vi "Autonomous Independent.vi"() -> ()   [LabVIEW 2015]
doc: "This VI is called when autonomous begins, and will automatically be terminated when autonomous ends. You can carry out timed or sensor driven robot movement independently without needing to return to the caller."
uses:
  <vilib>/Rock Robotics/WPI/Utilities/WPI_GetSetVariantRefNum.vi
  <vilib>/Rock Robotics/Network Tables/NT Write Numeric Array.vi
  <vilib>/Rock Robotics/Network Tables/NT Read Boolean.vi
  <vilib>/Rock Robotics/Network Tables/NT Write Boolean.vi
  <vilib>/Rock Robotics/Network Tables/NT Write Number.vi
  <vilib>/Rock Robotics/Network Tables/NT Read Number.vi
  <vilib>/Rock Robotics/WPI/RobotDrive/WPI_RobotDriveArcadeDrive_Standard(NoSaturation).vi
panel:
  in  "Ticks to Turn":i32=36
  out "VAR-Storage-1":dbl
  out "Low Switch":bool
  out "High Switch":bool
  out "POT Sensor Meter":dbl(knob) scale=78.0..98.0
  out "POT Sensor Value":dbl
  # "Remeber to Right Click:\nData Operatoins -> Make Current Value Default"
  # "Also This value is the \nTotal amount of ticks not Turns!\n\nSo 6 Ticks EQU 1 Full Turn."
  # "Be sure to right-click and choose Data Operations>>Make Current Value default if you want to save the array values with the VI"
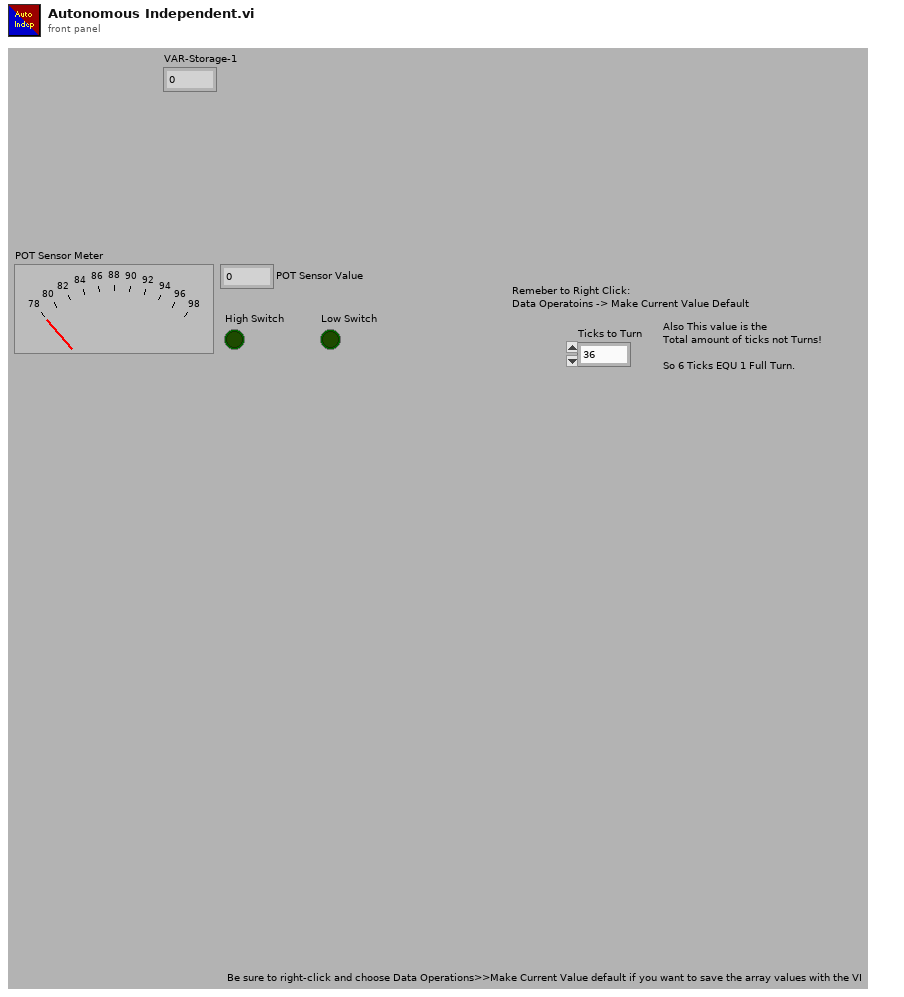
[diagram p1: front panel]
types:
  T1 = typedef "WPI_JoystickDevRef.ctl" = cluster{"Device":T2}
  T2 = typedef "WPI_JoystickDeviceEnum.ctl" = enum16{"USB 0", "USB 1", "USB 2", "USB 3", "USB 4", "USB 5"}
  T3 = typedef "WPI_CounterDevRef.ctl" = cluster{"DevStatus":errorcluster, "CntIndex":T4}
  T4 = typedef "FPGA_CounterCtrSystemIndex.ctl" = enum8{"Ctr 0", "Ctr 1", "Ctr 2", "Ctr 3", "Ctr 4", "Ctr 5", "Ctr 6", "Ctr 7", "Invalid"}
  T5 = typedef "WPI_SwitchDevRef.ctl" = cluster{"DevStatus":errorcluster, "DIO Channel":T6, "CntIndex":T4, "Normally Closed":bool}
  T6 = typedef "FPGA_DIOChannel.ctl" = enum8{"DIO 0", "DIO 1", "DIO 2", "DIO 3", "DIO 4", "DIO 5", "DIO 6", "DIO 7", "DIO 8", "DIO 9", "DIO MXP 0", "DIO MXP 1", "DIO MXP 2", "DIO MXP 3", "DIO MXP 4", "DIO MXP 5", "DIO MXP 6", "DIO MXP 7", "DIO MXP 8", "DIO MXP 9", "DIO MXP 10", "DIO MXP 11", "DIO MXP 12", "DIO MXP 13", "DIO MXP 14", "DIO MXP 15", "Invalid"}
  T7 = typedef "WPI_PotentiometerDevRef.ctl" = cluster{"DevStatus":errorcluster, "Analog Channel":T8, "Invert Output":bool}
  T8 = typedef "FPGA_AIChannel.ctl" = enum8{"AI 0", "AI 1", "AI 2", "AI 3", "AI MXP 0", "AI MXP 1", "AI MXP 2", "AI MXP 3", "Invalid"}
  T9 = typedef "WPI_MotorControlDeviceRef.ctl" = cluster{"DeviceStatus":errorcluster, "Type":T10, "PWM":cluster{"PWM Channel":T11, "DeadBand":T12}, "CAN":cluster{"Device Number":u8, "Control Mode":T13, "Semaphore":T14, "Max Vout":dbl, "TalonSRX Control Mode":T15}, "Invert":bool}
  T10 = typedef "WPI_MotorControlType.ctl" = enum16{"PWM", "CAN", "CANTalonSRX"}
  T11 = typedef "FPGA_DIOPWMChannel.ctl" = enum8{"PWM 0", "PWM 1", "PWM 2", "PWM 3", "PWM 4", "PWM 5", "PWM 6", "PWM 7", "PWM 8", "PWM 9", "PWM MXP 0", "PWM MXP 1", "PWM MXP 2", "PWM MXP 3", "PWM MXP 4", "PWM MXP 5", "PWM MXP 6", "PWM MXP 7", "PWM MXP 8", "PWM MXP 9", "Invalid"}
  T12 = typedef "WPI_PWMDeadband.ctl" = cluster{"Name":string, "maxPositivePwm":i32, "minPositivePwm":i32, "centerPwm":i32, "maxNegativePwm":i32, "minNegativePwm":i32, "angularRange":u16}
  T13 = typedef "WPI_CANJaguar_ControlMode.ctl" = enum8{"Percent VBus", "Current", "Speed", "Position", "Voltage"}
  T14 = typedef "Semaphore RefNum" = refnum<k1>
  T15 = typedef "WPI_CANTalonSRX_APIControlMode.ctl" = enum8{"Percent VBus", "Speed", "Position", "Slave", "Unchanged / Invalid", "Voltage Compensation", "Current", "Motion Profile"}
  T16 = typedef "WPI_RobotDriveDevRef.ctl" = cluster{"DevStatus":errorcluster, "Motors[]":T9[], "Square Inputs":bool, "Max Output":dbl}
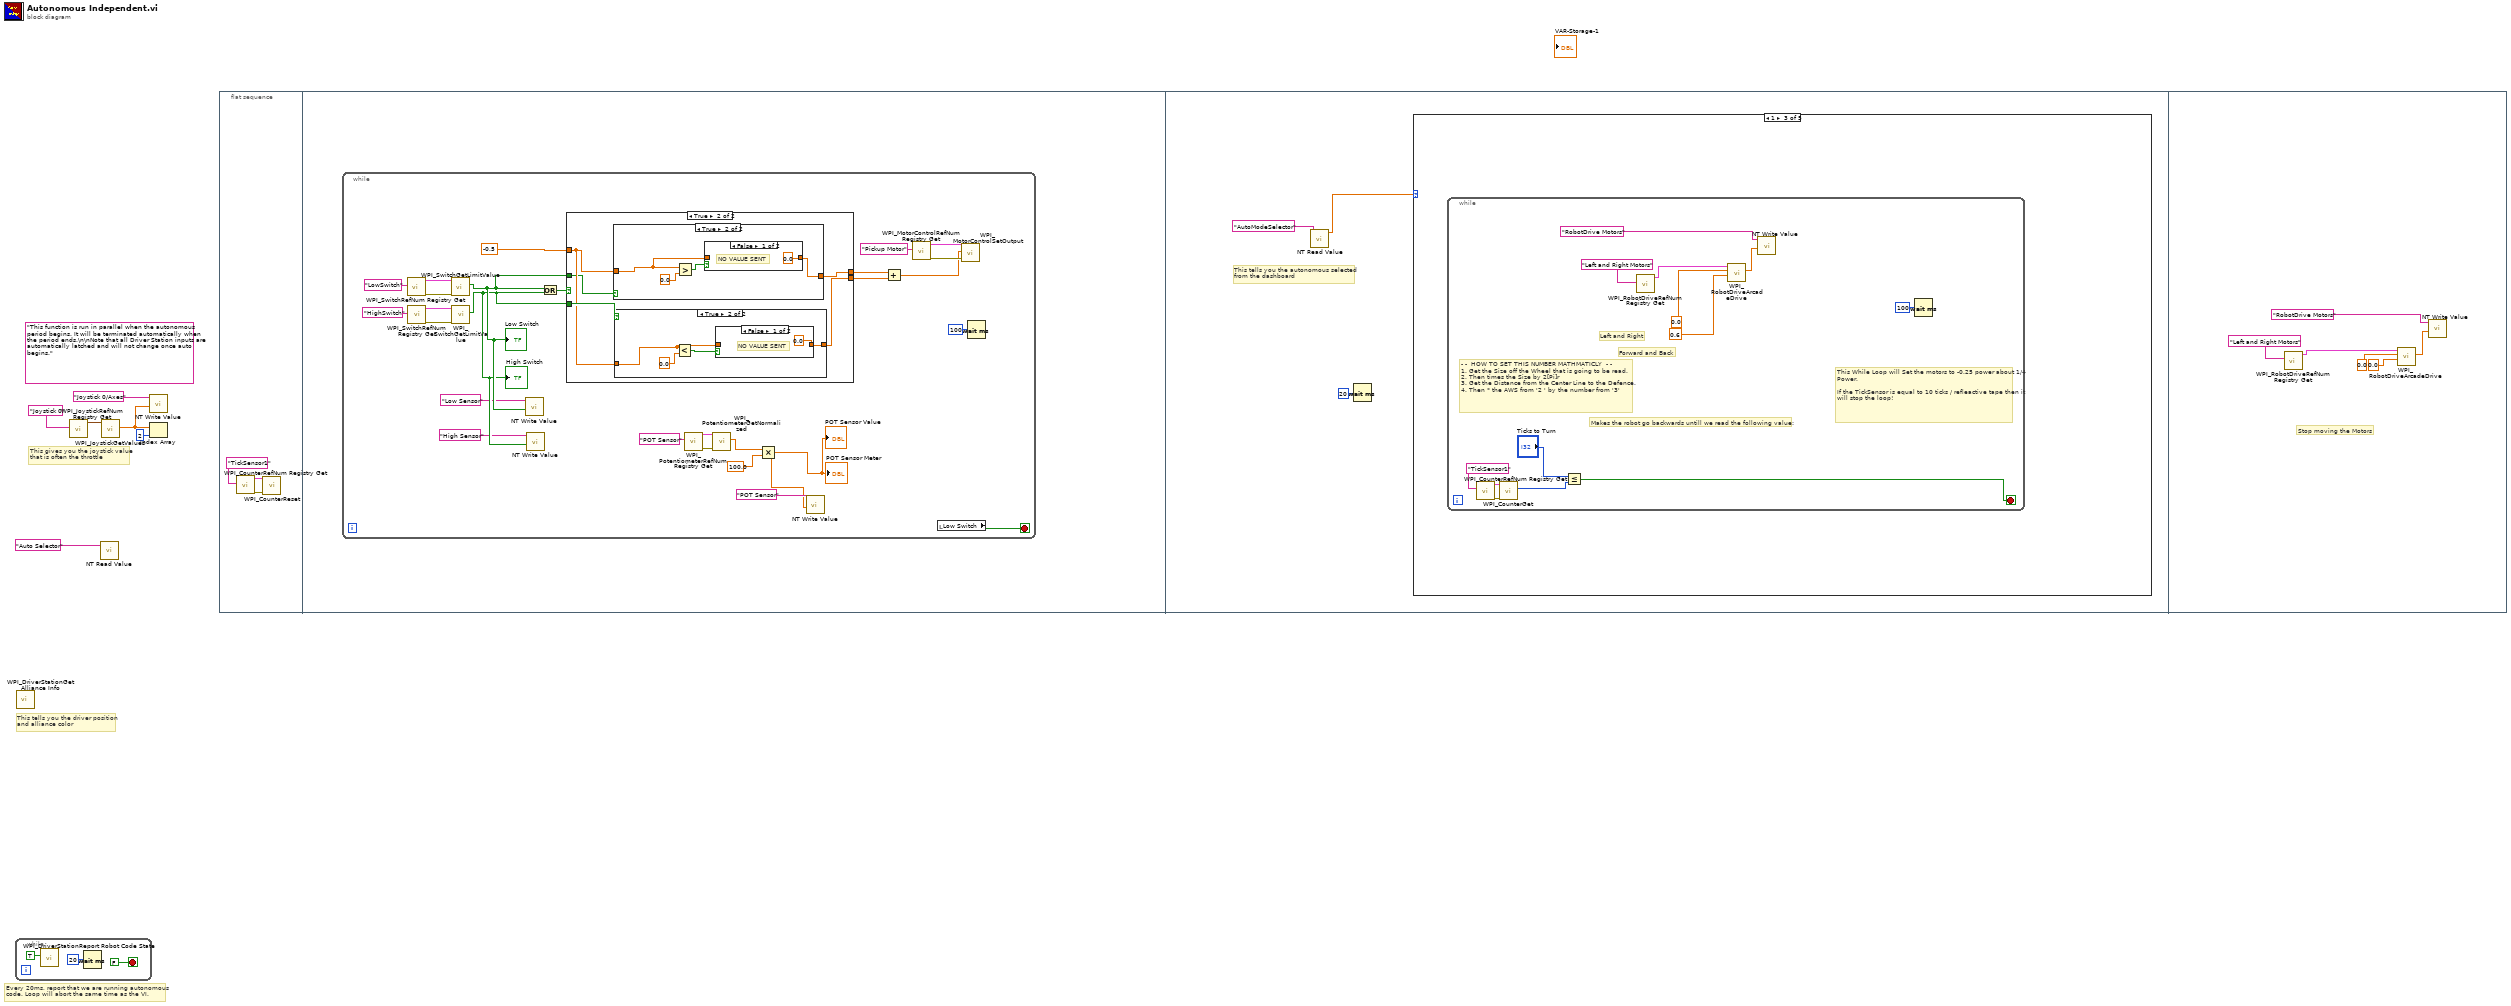
[diagram p0: block diagram]
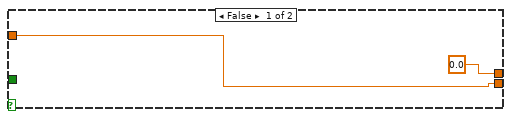
[diagram p2: hidden frame]
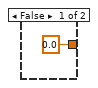
[diagram p3: hidden frame]
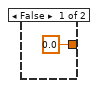
[diagram p5: hidden frame]
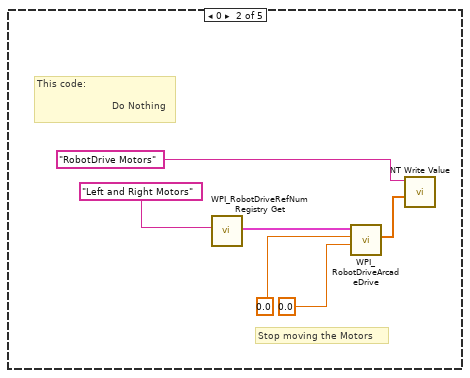
[diagram p8: hidden frame]
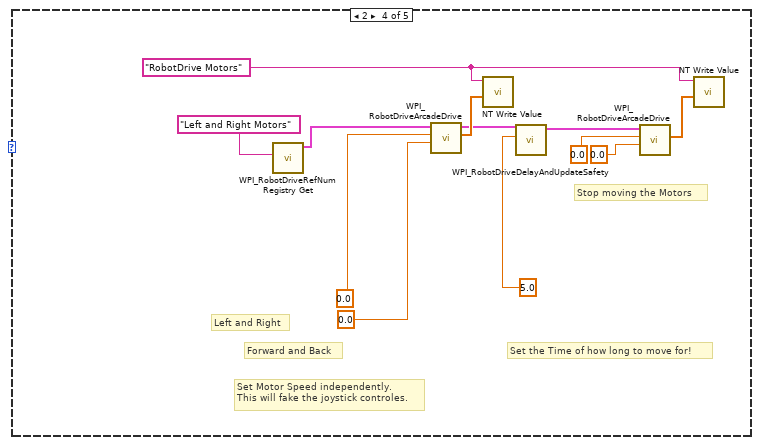
[diagram p9: hidden frame]
diagram:
  (unwired) "This function is run in parallel when the autonomous period begins. It will be terminated automatically when the period ends.\n\nNote that all Driver Station inputs are automatically latched and will not change once auto begins."
  # "Every 20ms, report that we are running autonomous\ncode. Loop will abort the same time as the VI."
  # "This gives you the joystick value\nthat is often the throttle"
  # "This tells you the driver position\nand alliance color"
  n1 = while {
    stop <- FALSE stop-if-true
    n2 = call <vilib>:"WPI_DriverStationReport Robot Code State.vi"("Autonomous"=TRUE) -> ()  [unwired: 10 in, 1 out]
    n3 = Wait (ms)(milliseconds to wait=u32 20) -> ()  [unwired: 1 out]
  }
  n4 = call <vilib>:"WPI_DriverStationGet Alliance Info.vi"() -> ()  [unwired: 12 out]
  n5 = call <vilib>:"WPI_JoystickRefNum Registry Get.vi"("refnum name"="Joystick 0") -> ("JoystickDevRef"=w5:T1)  [unwired: 1 in, 9 out]
  n6 = call-poly <vilib>:"NT Read Value.vi"("Name"="Auto Selector") -> ()  [unwired: 9 in, 2 out]
  n7 = call <vilib>:"WPI_JoystickGetValues.vi"("JoystickDevRef"=w5) -> ("Axes"=w3:dbl[])  [unwired: 6 in, 4 out]
  n8 = call-poly <vilib>:"NT Write Value.vi"("Numeric Array"=w3, "Name"="Joystick 0/Axes") -> ()  [unwired: 9 in, 1 out]
  n9 = Index Array(array=w3, index=2) -> ()  [unwired: 1 out]
  n10 = flat-sequence {
    frame #0 {
      n11 = call <vilib>:"WPI_CounterRefNum Registry Get.vi"("refnum name"="TickSensor1") -> ("error out"=w11:errorcluster, "CounterDevRef"=w10:T3)  [unwired: 9 in]
      n12 = call <vilib>:"WPI_CounterReset.vi"("error in (no error)"=w11, "CounterDevRef in"=w10) -> ()  [unwired: 8 in, 2 out]
    }
    frame #1 {
      n13 = while {
        stop <- w14 stop-if-true
        n14 = call <vilib>:"WPI_SwitchRefNum Registry Get.vi"("refnum name"="LowSwitch") -> ("error out"=w37:errorcluster, "SwitchDevRef"=w38:T5)  [unwired: 9 in]
        n15 = call <vilib>:"WPI_SwitchRefNum Registry Get.vi"("refnum name"="HighSwitch") -> ("error out"=w34:errorcluster, "SwitchDevRef"=w35:T5)  [unwired: 9 in]
        n16 = call <vilib>:"WPI_SwitchGetLimitValue.vi"("error in (no error)"=w37, "SwitchDevRef"=w38) -> ("Switch Pressed"=w22:bool)  [unwired: 7 in, 2 out]
        "Low Switch" <- w22
        n17 = call <vilib>:"WPI_SwitchGetLimitValue.vi"("error in (no error)"=w34, "SwitchDevRef"=w35) -> ("Switch Pressed"=w21:bool)  [unwired: 7 in, 2 out]
        "High Switch" <- w21
        n18 = call-poly <vilib>:"NT Write Value.vi"("Boolean"=w22, "Name"="Low Sensor") -> ()  [unwired: 9 in, 1 out]
        n19 = call-poly <vilib>:"NT Write Value.vi"("Boolean"=w21, "Name"="High Sensor") -> ()  [unwired: 9 in, 1 out]
        n20 = Or(x=w22, y=w21) -> (x .or. y?=w39:bool)
        n21 = case shown="True" w39 {
          tunnel: w22 -> [_ w44]
          tunnel: w21 -> [_ w46]
          tunnel: -0.5 ("Axes[1]") -> [w40 w45]
          tunnel: [0.0 ("Axes[1]") w43] -> w28
          tunnel: [w40 w42] -> w27
          frame False {
          }
          frame True {
            n22 = case shown="True" w44 {
              tunnel: w45 -> [_ w56]
              tunnel: [0.0 ("Axes[1]") w55] -> w43
              frame False {
              }
              frame True {
                n23 = Greater?(x=w56, y=0.0) -> (0:w57:bool)
                n24 = case shown="False" w57 {
                  tunnel: [0.0 ("Axes[1]") w60] -> w55
                  tunnel: w56 -> [_ w60]
                  frame False {
                    # "NO VALUE SENT"
                  }
                  frame True {
                  }
                }
              }
            }
            n25 = case shown="True" w46 {
              tunnel: w45 -> [_ w48]
              tunnel: [0.0 ("Axes[1]") w49] -> w42
              frame False {
              }
              frame True {
                n26 = Less?(x=w48, y=0.0) -> (x < y?=w50:bool)
                n27 = case shown="False" w50 {
                  tunnel: [0.0 ("Axes[1]") w53] -> w49
                  tunnel: w48 -> [_ w53]
                  frame False {
                    # "NO VALUE SENT"
                  }
                  frame True {
                  }
                }
              }
            }
          }
        }
        n28 = call <vilib>:"WPI_PotentiometerRefNum Registry Get.vi"("refnum name"="POT Sensor") -> ("error out"=w26:errorcluster, "PotDevRef"=w25:T7)  [unwired: 9 in]
        n29 = call <vilib>:"WPI_PotentiometerGetNormalized.vi"("error in"=w26, "PotDevRef"=w25) -> ("Normalized Value"=w18:dbl)  [unwired: 7 in, 2 out]
        n30 = Multiply(x=w18, y=100.0) -> (x*y=w16:dbl)
        "POT Sensor Value" <- w16
        "POT Sensor Meter" <- w16
        n31 = call-poly <vilib>:"NT Write Value.vi"("Numeric"=w16, "Name"="POT Sensor") -> ()  [unwired: 9 in, 1 out]
        n32 = Add(x=w28, y=w27) -> (x+y=w29:dbl)
        n33 = call <vilib>:"WPI_MotorControlRefNum Registry Get.vi"("refnum name"="Pickup Motor") -> ("error out"=w32:errorcluster, "MotorControlDevRef"=w31:T9)  [unwired: 9 in]
        n34 = local read "Low Switch"() -> (w14:bool)
        n35 = call <vilib>:"WPI_MotorControlSetOutput.vi"("error in (no error)"=w32, "Output"=w29, "MotorControlDevRef"=w31) -> ()  [unwired: 6 in, 3 out]
        n36 = Wait (ms)(milliseconds to wait=u32 100) -> ()  [unwired: 1 out]
      }
    }
    frame #2 {
      # "This tells you the autonomous selected\nfrom the dashboard"
      n37 = call-poly <vilib>:"NT Read Value.vi"("Name"="AutoModeSelector") -> ("Numeric"=w62:dbl)  [unwired: 9 in, 1 out]
      n38 = Wait (ms)(milliseconds to wait=u32 20) -> ()  [unwired: 1 out]
      n39 = case shown="1" w62 {
        frame Default {
          # "You can put your main auto here, or you can right-click on the case and make any\nother frame be the default case."
          # "This is the frame that will execute if no selection is made, or if it is not recognized"
        }
        frame 0 {
          # "Stop moving the Motors"
          # "This code:\n                   \n                         Do Nothing"
          n40 = call <vilib>:"WPI_RobotDriveRefNum Registry Get.vi"("refnum name"="Left and Right Motors") -> ("RobotDriveDevRef"=w64:T16)  [unwired: 1 in, 9 out]
          n41 = call-poly <vilib>:"WPI_RobotDriveArcadeDrive.vi"("Y axis value"=0.0 ("X axis value"), "X axis value"=0.0, "RobotDriveDevRef"=w64) -> ("Motor Values"=w68:dbl[])  [unwired: 1 in, 7 out]
          n42 = call-poly <vilib>:"NT Write Value.vi"("Numeric Array"=w68, "Name"="RobotDrive Motors") -> ()  [unwired: 9 in, 1 out]
        }
        frame 1 {
          n43 = while {
            stop <- w79 stop-if-true
            # "- -  HOW TO SET THIS NUMBER MATHMATICLY  - - \n1. Get the Size off the Wheel that is going to be read.\n2. Then times the Size by 2[Pi]r\n3. Get the Distance from the Center Line to the Defence.\n4. Then * the AWS from '2 ' by the number from '3'"
            # "Makes the robot go backwards untill we read the following value:"
            # "This While Loop will Set the motors to -0.25 power about 1/4 Power.\n\nIf the TickSensor is equal to 10 ticks / refleactive tape then it will stop the loop!"
            # "Forward and Back"
            # "Left and Right"
            n44 = call <vilib>:"WPI_CounterRefNum Registry Get.vi"("refnum name"="TickSensor1") -> ("error out"=w81:errorcluster, "CounterDevRef"=w80:T3)  [unwired: 9 in]
            n45 = call <vilib>:"WPI_CounterGet.vi"("error in (no error)"=w81, "CounterDevRef in"=w80) -> ("Value"=w71:i32)  [unwired: 4 in, 5 out]
            n46 = Less Or Equal?(x="Ticks to Turn", y=w71) -> (x <= y?=w79:bool)
            n47 = call <vilib>:"WPI_RobotDriveRefNum Registry Get.vi"("refnum name"="Left and Right Motors") -> ("RobotDriveDevRef"=w78:T16)  [unwired: 1 in, 9 out]
            n48 = call-poly <vilib>:"WPI_RobotDriveArcadeDrive.vi"("Y axis value"=0.6 ("X axis value"), "X axis value"=0.0, "RobotDriveDevRef"=w78) -> ("Motor Values"=w76:dbl[])  [unwired: 1 in, 7 out]
            n49 = call-poly <vilib>:"NT Write Value.vi"("Numeric Array"=w76, "Name"="RobotDrive Motors") -> ()  [unwired: 9 in, 1 out]
            n50 = Wait (ms)(milliseconds to wait=u32 100) -> ()  [unwired: 1 out]
          }
        }
        frame 2 {
          w93 = "RobotDrive Motors" ("Name")
          # "Forward and Back"
          # "Left and Right"
          # "Set Motor Speed independently.\nThis will fake the joystick controles."
          # "Set the Time of how long to move for!"
          # "Stop moving the Motors"
          n51 = call <vilib>:"WPI_RobotDriveRefNum Registry Get.vi"("refnum name"="Left and Right Motors") -> ("RobotDriveDevRef"=w94:T16)  [unwired: 1 in, 9 out]
          n52 = call-poly <vilib>:"WPI_RobotDriveArcadeDrive.vi"("Y axis value"=0.0 ("X axis value"), "X axis value"=0.0, "RobotDriveDevRef"=w94) -> ("Motor Values"=w92:dbl[], "RobotDriveDevRef"=w86:T16)  [unwired: 1 in, 6 out]
          n53 = call-poly <vilib>:"NT Write Value.vi"("Numeric Array"=w92, "Name"=w93) -> ()  [unwired: 9 in, 1 out]
          n54 = call <vilib>:"WPI_RobotDriveDelayAndUpdateSafety.vi"("Delay (s)"=5.0, "RobotDriveDevRef"=w86) -> ("RobotDriveDevRef 2"=w85:T16)  [unwired: 8 in, 1 out]
          n55 = call-poly <vilib>:"WPI_RobotDriveArcadeDrive.vi"("Y axis value"=0.0 ("X axis value"), "X axis value"=0.0, "RobotDriveDevRef"=w85) -> ("Motor Values"=w91:dbl[])  [unwired: 1 in, 7 out]
          n56 = call-poly <vilib>:"NT Write Value.vi"("Numeric Array"=w91, "Name"=w93) -> ()  [unwired: 9 in, 1 out]
        }
        frame 3 {
        }
      }
    }
    frame #3 {
      # "Stop moving the Motors"
      n57 = call <vilib>:"WPI_RobotDriveRefNum Registry Get.vi"("refnum name"="Left and Right Motors") -> ("RobotDriveDevRef"=w95:T16)  [unwired: 1 in, 9 out]
      n58 = call-poly <vilib>:"WPI_RobotDriveArcadeDrive.vi"("Y axis value"=0.0 ("X axis value"), "X axis value"=0.0, "RobotDriveDevRef"=w95) -> ("Motor Values"=w97:dbl[])  [unwired: 1 in, 7 out]
      n59 = call-poly <vilib>:"NT Write Value.vi"("Numeric Array"=w97, "Name"="RobotDrive Motors") -> ()  [unwired: 9 in, 1 out]
    }
  }
